vi "Verify SICK Data.vi"(1 "SICK Data":T1) -> (0 "Data OK?":bool)   [LabVIEW 2009]
uses:
  TypeDefs/Sensor Typedefs/SICK Array.ctl
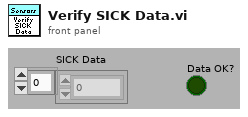
[diagram p1: front panel]
types:
  T1 = typedef "SICK Array.ctl" = u16[]
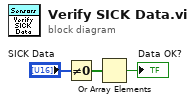
[diagram p0: block diagram]
diagram:
  n1 = Not Equal To 0?(x="SICK Data") -> (x != 0?=w2:bool[])
  n2 = Or Array Elements(Boolean array=w2) -> (logical OR=→"Data OK?":bool)
